vi "Initialise.vi"(8 "error in (no error)":errorcluster, 10 "System In":refnum<class "abs_System.lvclass">, 11 "Node in":refnum<class "abs_Decorator.lvclass">) -> (0 "error out":errorcluster, 2 "System Out":refnum<class "abs_System.lvclass">, 3 "Node out":refnum<class "abs_Decorator.lvclass">)   [LabVIEW 2021, in "BT.lvlib" / "abs_Decorator.lvclass"]
uses:
  abs_Decorator.lvclass
  abs_System/abs_System.lvclass
  abs_Decorator.lvclass/abs_Decorator.ctl
  abs_Node/abs_Node.lvclass
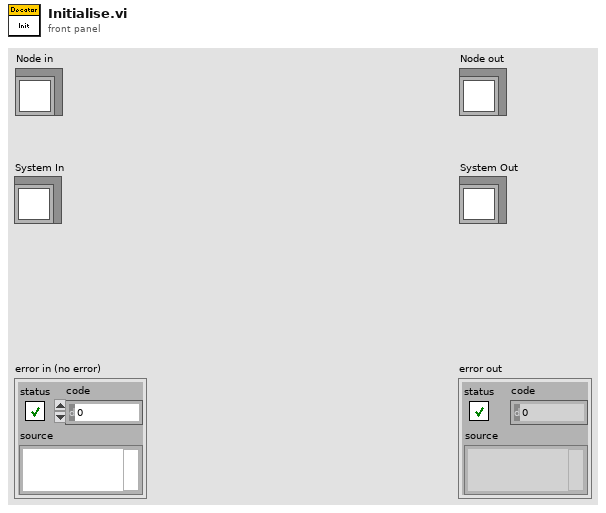
[diagram p1: front panel]
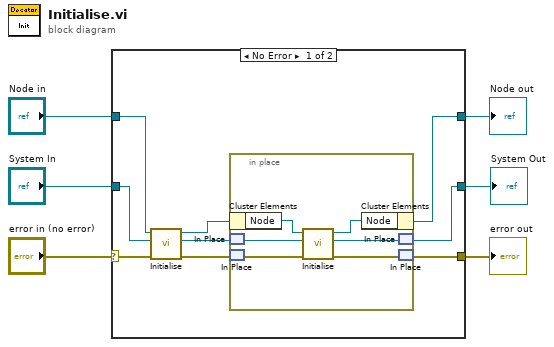
[diagram p0: block diagram]
diagram:
  n1 = case shown="No Error" "error in (no error)" {
    selector: "error in (no error)" -> [w15 w22]
    tunnel: "System In" -> [w14 w23]
    tunnel: "Node in" -> [w13 w24]
    tunnel: [w11 w24] -> w3
    tunnel: [w8 w22] -> w2
    tunnel: [w7 w23] -> w1
    frame No Error {
      n2 = call-parent "Initialise.vi"("error in (no error)"=w15, "System In"=w14, "Node in"=w13) -> ("error out"=w9:errorcluster, "System Out"=w10:refnum<class "abs_System.lvclass">, "Node out"=w12:refnum<class "abs_Decorator.lvclass">)  [unwired: 6 in]
      n3 = in-place {
        n4 = in-place-cluster #1(w12) -> ("Node"=w21:refnum<class "abs_Node.lvclass">)
        n5 = in-place-match #2(w10) -> (w19:refnum<class "abs_System.lvclass">)
        n6 = in-place-match #3(w9) -> (w17:errorcluster)
        n7 = call-dynamic "Initialise.vi"("error in (no error)"=w17, "System In"=w19, "Node in"=w21) -> ("error out"=w16:errorcluster, "System Out"=w18:refnum<class "abs_System.lvclass">, "Node out"=w20:refnum<class "abs_Node.lvclass">)  [unwired: 6 in]
        n8 = in-place-cluster #1("Node"=w20) -> (w11:refnum<class "abs_Decorator.lvclass">)
        n9 = in-place-match #2(w18) -> (w7:refnum<class "abs_System.lvclass">)
        n10 = in-place-match #3(w16) -> (w8:errorcluster)
      }
    }
    frame Error {
    }
  }
  "error out" <- w2
  "Node out" <- w3
  "System Out" <- w1
